vi "Write AckTime.vi"(8 "error in (no error)":errorcluster, 10 "AckTime":timestamp, 11 "Request in":refnum<class "Request.lvclass">) -> (0 "error out":errorcluster, 3 "Request out":refnum<class "Request.lvclass">)   [LabVIEW 2015, in "Request.lvclass"]
uses:
  Request.lvclass
  Request.lvclass/Request.ctl
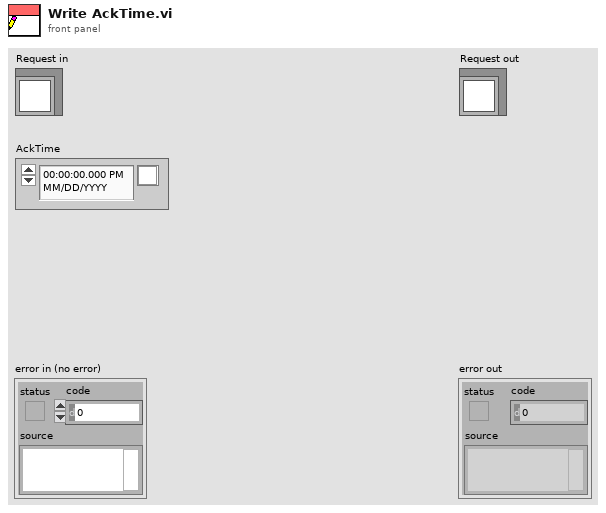
[diagram p1: front panel]
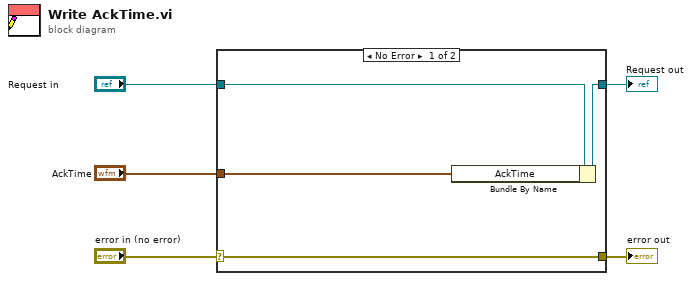
[diagram p0: block diagram]
diagram:
  n1 = case shown="No Error" "error in (no error)" {
    selector: "error in (no error)" -> [w9 w10]
    tunnel: [w9 w10] -> w4
    tunnel: [w7 w11] -> w2
    tunnel: "Request in" -> [w8 w11]
    tunnel: "AckTime" -> [w6 _]
    frame No Error {
      n2 = Bundle By Name(cluster=w8, "AckTime"=w6) -> (w7:refnum<class "Request.lvclass">)
    }
    frame Error {
    }
  }
  "error out" <- w4
  "Request out" <- w2
